vi "calculate CO.vi"() -> ()   [LabVIEW 2023]
uses:
  <vilib>/Utility/file.llb/Read Delimited Spreadsheet (DBL).vi
panel:
  out "Waveform Graph":dbl[](graph)
  out "mean CO recovery":dbl
  out "CO recovery":dbl[](array[numeric])
  out "mean CO stage4":dbl
  out "CO stage4":dbl[](array[numeric])
  out "mean CO stage3":dbl
  out "CO stage3":dbl[](array[numeric])
  out "mean CO stage2":dbl
  out "CO stage2":dbl[](array[numeric])
  out "mean CO stage1":dbl
  out "CO stage1":dbl[](array[numeric])
  out "mean CO baseline":dbl
  out "CO baseline":dbl[](array[numeric])
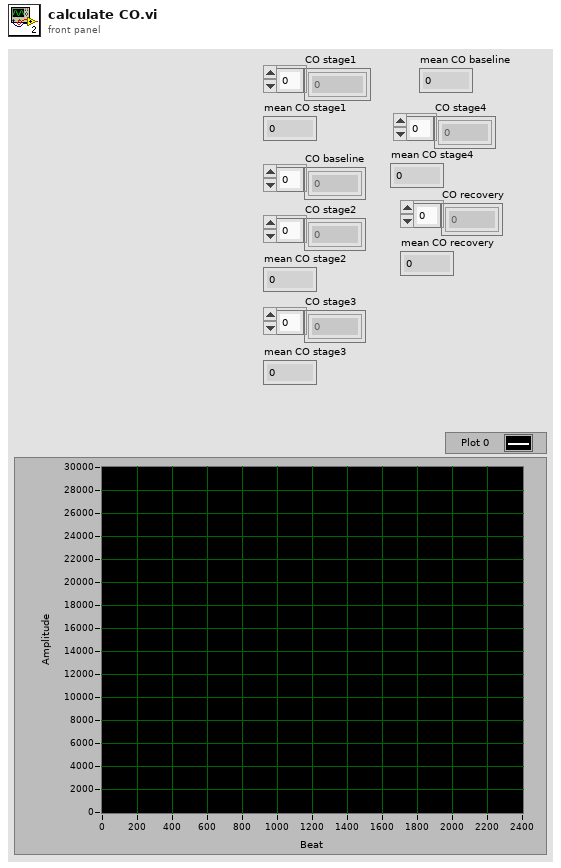
[diagram p1: front panel]
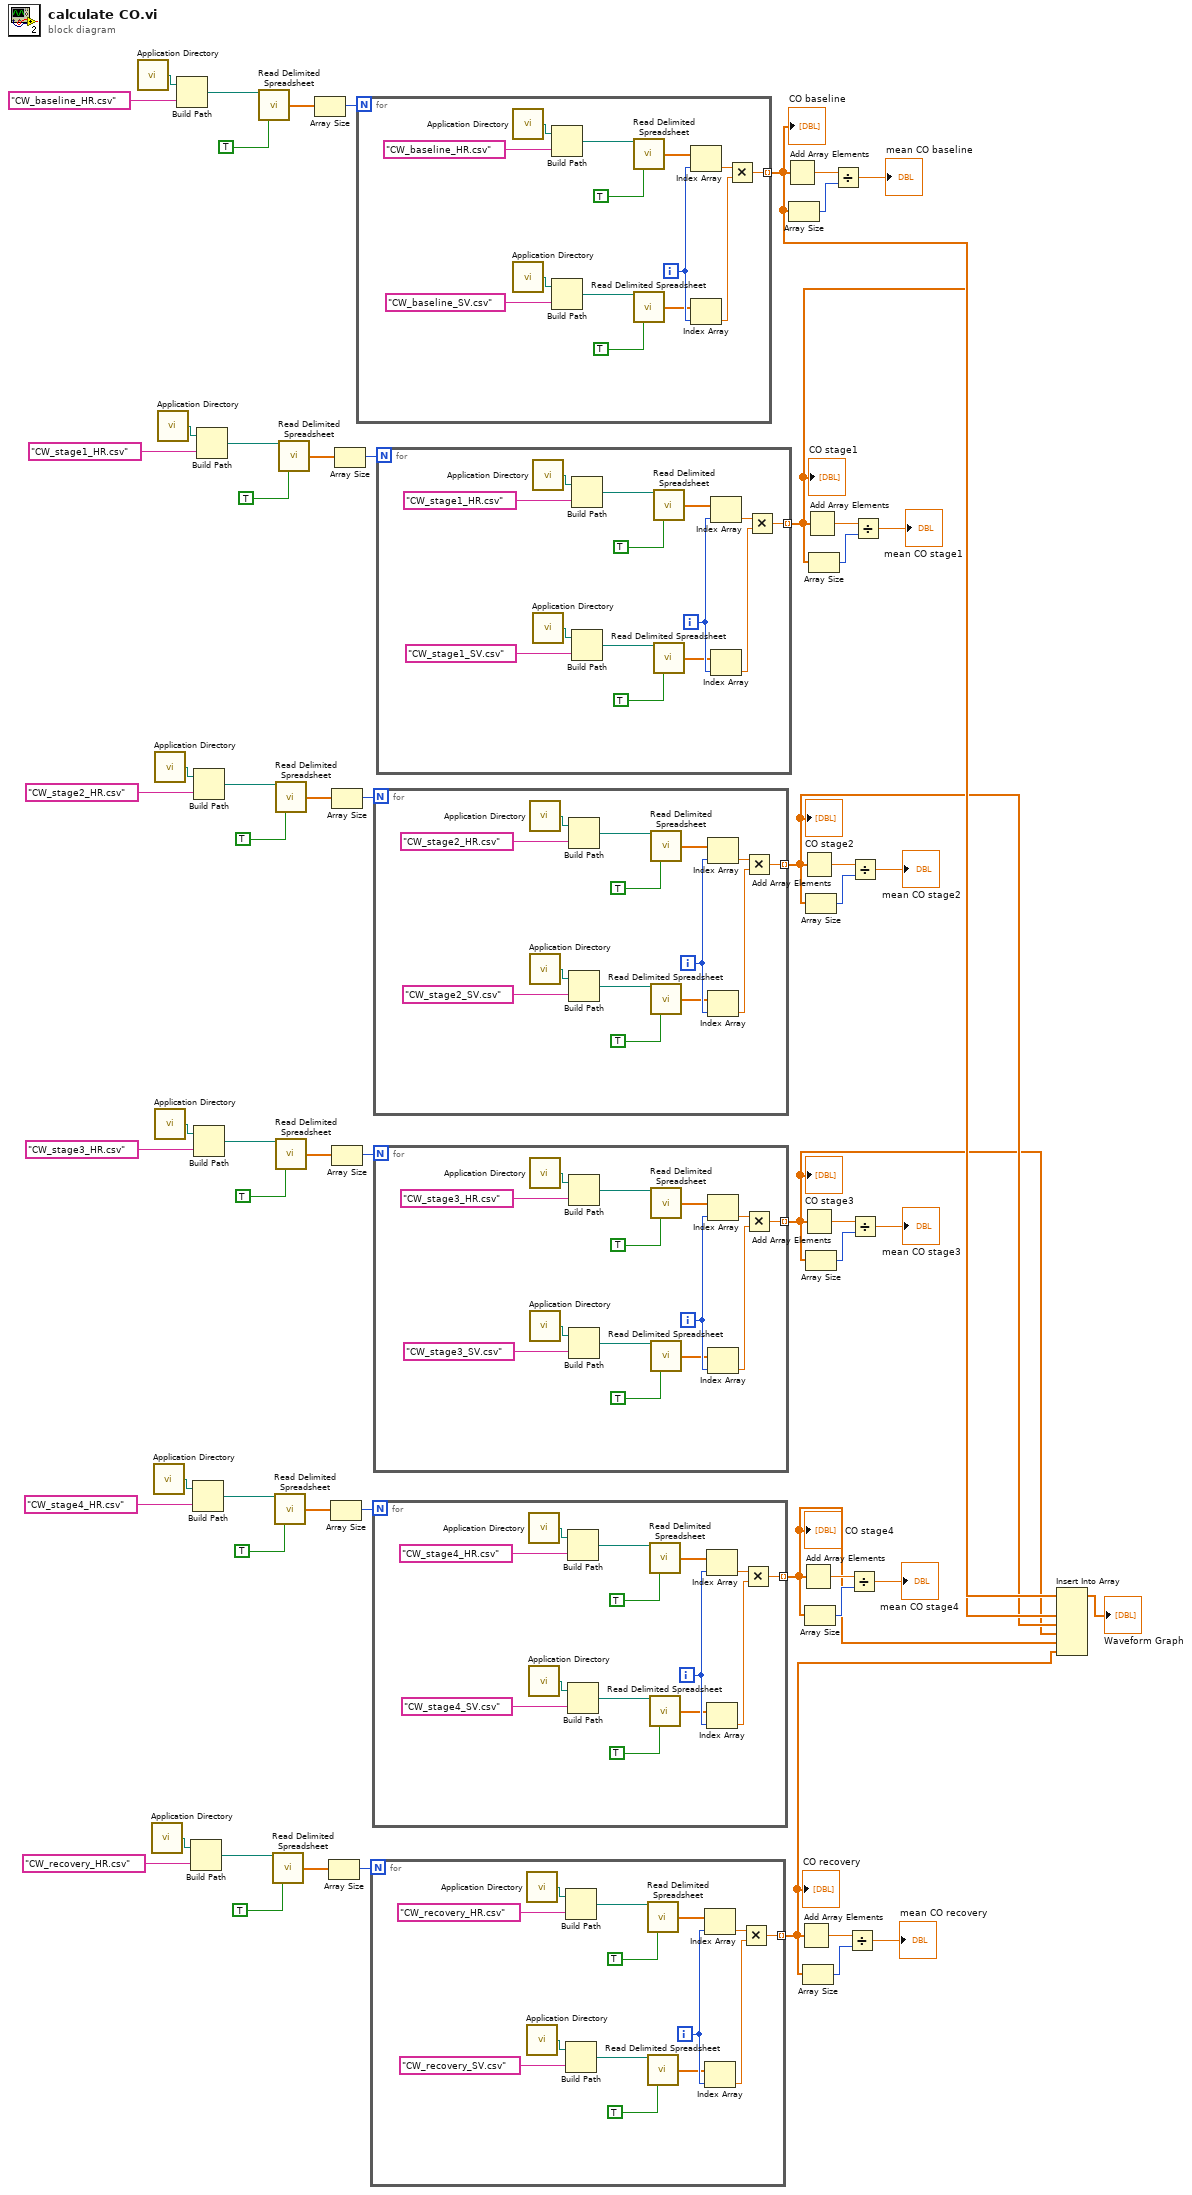
[diagram p0: block diagram]
diagram:
  n1 = call <vilib>:"Application Directory.vi"() -> ("Application Directory"=w57:path)
  n2 = call <vilib>:"Application Directory.vi"() -> ("Application Directory"=w12:path)
  n3 = call <vilib>:"Application Directory.vi"() -> ("Application Directory"=w21:path)
  n4 = call <vilib>:"Application Directory.vi"() -> ("Application Directory"=w39:path)
  n5 = call <vilib>:"Application Directory.vi"() -> ("Application Directory"=w30:path)
  n6 = call <vilib>:"Application Directory.vi"() -> ("Application Directory"=w48:path)
  n7 = Build Path(base path=w57, name or relative path="CW_baseline_HR.csv") -> (appended path=w54:path)
  n8 = Build Path(base path=w12, name or relative path="CW_recovery_HR.csv") -> (appended path=w9:path)
  n9 = Build Path(base path=w21, name or relative path="CW_stage4_HR.csv") -> (appended path=w18:path)
  n10 = Build Path(base path=w39, name or relative path="CW_stage2_HR.csv") -> (appended path=w36:path)
  n11 = Build Path(base path=w30, name or relative path="CW_stage3_HR.csv") -> (appended path=w27:path)
  n12 = Build Path(base path=w48, name or relative path="CW_stage1_HR.csv") -> (appended path=w45:path)
  n13 = call-poly <vilib>:"Read Delimited Spreadsheet.vi"("file path (dialog if empty)"=w54, "transpose? (F)"=TRUE) -> ("first row"=w53:dbl[])  [unwired: 8 in, 5 out]
  n14 = call-poly <vilib>:"Read Delimited Spreadsheet.vi"("file path (dialog if empty)"=w9, "transpose? (F)"=TRUE) -> ("first row"=w8:dbl[])  [unwired: 8 in, 5 out]
  n15 = call-poly <vilib>:"Read Delimited Spreadsheet.vi"("file path (dialog if empty)"=w18, "transpose? (F)"=TRUE) -> ("first row"=w17:dbl[])  [unwired: 8 in, 5 out]
  n16 = call-poly <vilib>:"Read Delimited Spreadsheet.vi"("file path (dialog if empty)"=w36, "transpose? (F)"=TRUE) -> ("first row"=w35:dbl[])  [unwired: 8 in, 5 out]
  n17 = call-poly <vilib>:"Read Delimited Spreadsheet.vi"("file path (dialog if empty)"=w27, "transpose? (F)"=TRUE) -> ("first row"=w26:dbl[])  [unwired: 8 in, 5 out]
  n18 = call-poly <vilib>:"Read Delimited Spreadsheet.vi"("file path (dialog if empty)"=w45, "transpose? (F)"=TRUE) -> ("first row"=w44:dbl[])  [unwired: 8 in, 5 out]
  n19 = Array Size(array=w53) -> (size(s)=w61:i32)
  n20 = Array Size(array=w8) -> (size(s)=w16:i32)
  n21 = Array Size(array=w17) -> (size(s)=w25:i32)
  n22 = Array Size(array=w35) -> (size(s)=w43:i32)
  n23 = Array Size(array=w26) -> (size(s)=w34:i32)
  n24 = Array Size(array=w44) -> (size(s)=w52:i32)
  n25 = for {
    N: w61 -> [_]
    tunnel: [w74] -> w7 mode=indexing
    i -> [w75]
    n26 = call <vilib>:"Application Directory.vi"() -> ("Application Directory"=w73:path)
    n27 = call <vilib>:"Application Directory.vi"() -> ("Application Directory"=w68:path)
    n28 = Build Path(base path=w73, name or relative path="CW_baseline_HR.csv") -> (appended path=w70:path)
    n29 = Build Path(base path=w68, name or relative path="CW_baseline_SV.csv") -> (appended path=w65:path)
    n30 = call-poly <vilib>:"Read Delimited Spreadsheet.vi"("file path (dialog if empty)"=w70, "transpose? (F)"=TRUE) -> ("first row"=w69:dbl[])  [unwired: 8 in, 5 out]
    n31 = call-poly <vilib>:"Read Delimited Spreadsheet.vi"("file path (dialog if empty)"=w65, "transpose? (F)"=TRUE) -> ("first row"=w64:dbl[])  [unwired: 8 in, 5 out]
    n32 = Index Array(array=w69, index=w75) -> (element=w63:dbl)
    n33 = Index Array(array=w64, index=w75) -> (element=w62:dbl)
    n34 = Multiply(x=w63, y=w62) -> (x*y=w74:dbl)
  }
  "CO baseline" <- w7
  n35 = for {
    N: w16 -> [_]
    tunnel: [w88] -> w2 mode=indexing
    i -> [w89]
    n36 = call <vilib>:"Application Directory.vi"() -> ("Application Directory"=w87:path)
    n37 = call <vilib>:"Application Directory.vi"() -> ("Application Directory"=w82:path)
    n38 = Build Path(base path=w87, name or relative path="CW_recovery_HR.csv") -> (appended path=w84:path)
    n39 = Build Path(base path=w82, name or relative path="CW_recovery_SV.csv") -> (appended path=w79:path)
    n40 = call-poly <vilib>:"Read Delimited Spreadsheet.vi"("file path (dialog if empty)"=w84, "transpose? (F)"=TRUE) -> ("first row"=w83:dbl[])  [unwired: 8 in, 5 out]
    n41 = call-poly <vilib>:"Read Delimited Spreadsheet.vi"("file path (dialog if empty)"=w79, "transpose? (F)"=TRUE) -> ("first row"=w78:dbl[])  [unwired: 8 in, 5 out]
    n42 = Index Array(array=w83, index=w89) -> (element=w77:dbl)
    n43 = Index Array(array=w78, index=w89) -> (element=w76:dbl)
    n44 = Multiply(x=w77, y=w76) -> (x*y=w88:dbl)
  }
  "CO recovery" <- w2
  n45 = for {
    N: w25 -> [_]
    tunnel: [w102] -> w3 mode=indexing
    i -> [w103]
    n46 = call <vilib>:"Application Directory.vi"() -> ("Application Directory"=w101:path)
    n47 = call <vilib>:"Application Directory.vi"() -> ("Application Directory"=w96:path)
    n48 = Build Path(base path=w101, name or relative path="CW_stage4_HR.csv") -> (appended path=w98:path)
    n49 = Build Path(base path=w96, name or relative path="CW_stage4_SV.csv") -> (appended path=w93:path)
    n50 = call-poly <vilib>:"Read Delimited Spreadsheet.vi"("file path (dialog if empty)"=w98, "transpose? (F)"=TRUE) -> ("first row"=w97:dbl[])  [unwired: 8 in, 5 out]
    n51 = call-poly <vilib>:"Read Delimited Spreadsheet.vi"("file path (dialog if empty)"=w93, "transpose? (F)"=TRUE) -> ("first row"=w92:dbl[])  [unwired: 8 in, 5 out]
    n52 = Index Array(array=w97, index=w103) -> (element=w91:dbl)
    n53 = Index Array(array=w92, index=w103) -> (element=w90:dbl)
    n54 = Multiply(x=w91, y=w90) -> (x*y=w102:dbl)
  }
  "CO stage4" <- w3
  n55 = for {
    N: w43 -> [_]
    tunnel: [w116] -> w5 mode=indexing
    i -> [w117]
    n56 = call <vilib>:"Application Directory.vi"() -> ("Application Directory"=w115:path)
    n57 = call <vilib>:"Application Directory.vi"() -> ("Application Directory"=w110:path)
    n58 = Build Path(base path=w115, name or relative path="CW_stage2_HR.csv") -> (appended path=w112:path)
    n59 = Build Path(base path=w110, name or relative path="CW_stage2_SV.csv") -> (appended path=w107:path)
    n60 = call-poly <vilib>:"Read Delimited Spreadsheet.vi"("file path (dialog if empty)"=w112, "transpose? (F)"=TRUE) -> ("first row"=w111:dbl[])  [unwired: 8 in, 5 out]
    n61 = call-poly <vilib>:"Read Delimited Spreadsheet.vi"("file path (dialog if empty)"=w107, "transpose? (F)"=TRUE) -> ("first row"=w106:dbl[])  [unwired: 8 in, 5 out]
    n62 = Index Array(array=w111, index=w117) -> (element=w105:dbl)
    n63 = Index Array(array=w106, index=w117) -> (element=w104:dbl)
    n64 = Multiply(x=w105, y=w104) -> (x*y=w116:dbl)
  }
  "CO stage2" <- w5
  n65 = for {
    N: w34 -> [_]
    tunnel: [w130] -> w4 mode=indexing
    i -> [w131]
    n66 = call <vilib>:"Application Directory.vi"() -> ("Application Directory"=w129:path)
    n67 = call <vilib>:"Application Directory.vi"() -> ("Application Directory"=w124:path)
    n68 = Build Path(base path=w129, name or relative path="CW_stage3_HR.csv") -> (appended path=w126:path)
    n69 = Build Path(base path=w124, name or relative path="CW_stage3_SV.csv") -> (appended path=w121:path)
    n70 = call-poly <vilib>:"Read Delimited Spreadsheet.vi"("file path (dialog if empty)"=w126, "transpose? (F)"=TRUE) -> ("first row"=w125:dbl[])  [unwired: 8 in, 5 out]
    n71 = call-poly <vilib>:"Read Delimited Spreadsheet.vi"("file path (dialog if empty)"=w121, "transpose? (F)"=TRUE) -> ("first row"=w120:dbl[])  [unwired: 8 in, 5 out]
    n72 = Index Array(array=w125, index=w131) -> (element=w119:dbl)
    n73 = Index Array(array=w120, index=w131) -> (element=w118:dbl)
    n74 = Multiply(x=w119, y=w118) -> (x*y=w130:dbl)
  }
  "CO stage3" <- w4
  n75 = for {
    N: w52 -> [_]
    tunnel: [w144] -> w6 mode=indexing
    i -> [w145]
    n76 = call <vilib>:"Application Directory.vi"() -> ("Application Directory"=w143:path)
    n77 = call <vilib>:"Application Directory.vi"() -> ("Application Directory"=w138:path)
    n78 = Build Path(base path=w143, name or relative path="CW_stage1_HR.csv") -> (appended path=w140:path)
    n79 = Build Path(base path=w138, name or relative path="CW_stage1_SV.csv") -> (appended path=w135:path)
    n80 = call-poly <vilib>:"Read Delimited Spreadsheet.vi"("file path (dialog if empty)"=w140, "transpose? (F)"=TRUE) -> ("first row"=w139:dbl[])  [unwired: 8 in, 5 out]
    n81 = call-poly <vilib>:"Read Delimited Spreadsheet.vi"("file path (dialog if empty)"=w135, "transpose? (F)"=TRUE) -> ("first row"=w134:dbl[])  [unwired: 8 in, 5 out]
    n82 = Index Array(array=w139, index=w145) -> (element=w133:dbl)
    n83 = Index Array(array=w134, index=w145) -> (element=w132:dbl)
    n84 = Multiply(x=w133, y=w132) -> (x*y=w144:dbl)
  }
  "CO stage1" <- w6
  n85 = Add Array Elements(numeric array=w7) -> (sum=w59:dbl)
  n86 = Array Size(array=w7) -> (size(s)=w60:i32)
  n87 = Add Array Elements(numeric array=w2) -> (sum=w14:dbl)
  n88 = Add Array Elements(numeric array=w3) -> (sum=w23:dbl)
  n89 = Array Size(array=w2) -> (size(s)=w15:i32)
  n90 = Add Array Elements(numeric array=w5) -> (sum=w41:dbl)
  n91 = Add Array Elements(numeric array=w4) -> (sum=w32:dbl)
  n92 = Array Size(array=w3) -> (size(s)=w24:i32)
  n93 = Array Size(array=w5) -> (size(s)=w42:i32)
  n94 = Array Size(array=w4) -> (size(s)=w33:i32)
  n95 = Add Array Elements(numeric array=w6) -> (sum=w50:dbl)
  n96 = Array Size(array=w6) -> (size(s)=w51:i32)
  n97 = Divide(x=w59, y=w60) -> (x/y=→"mean CO baseline":dbl)
  n98 = Divide(x=w14, y=w15) -> (x/y=→"mean CO recovery":dbl)
  n99 = Divide(x=w23, y=w24) -> (x/y=→"mean CO stage4":dbl)
  n100 = Divide(x=w41, y=w42) -> (x/y=→"mean CO stage2":dbl)
  n101 = Divide(x=w32, y=w33) -> (x/y=→"mean CO stage3":dbl)
  n102 = Divide(x=w50, y=w51) -> (x/y=→"mean CO stage1":dbl)
  n103 = Insert Into Array(array=w7, new element #1=w6, new element #2=w5, new element #3=w4, new element #4=w3, new element #5=w2) -> (→"Waveform Graph":dbl[])  [unwired: 1 in]
